vi "_DRIVER_SHARED_INI_GenerateByDriverConnectorPane.vi"() -> ()   [LabVIEW 2020]
doc: "Generate File \"_HW-Configuration_.ini\" by file [...]_driver.vi This generate the INPUT SUBSECTION using controls linked in connector pane."
uses:
  TYPEDEF/_DRIVER_SHARED_TYPEDEF_INI-Method.ctl
panel:
  in  "Path of [...]_driver.vi":path=path "C:/UG-WORK/_DRIVER_/LV2020/NI9205/NI9205_driver.vi"
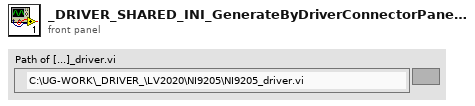
[diagram p1: front panel]
types:
  T1 = typedef "_DRIVER_SHARED_TYPEDEF_INI-Method.ctl" = enum16{"OPEN/CREATE", "READ", "WRITE", "CLOSE", "NO_OP"}
  T2 = typedef "_DRIVER_SHARED_TYPEDEF_StringControlVaviables.ctl" = cluster{"Ctrl Var Name":string, "String Ctrl Var Value":string}
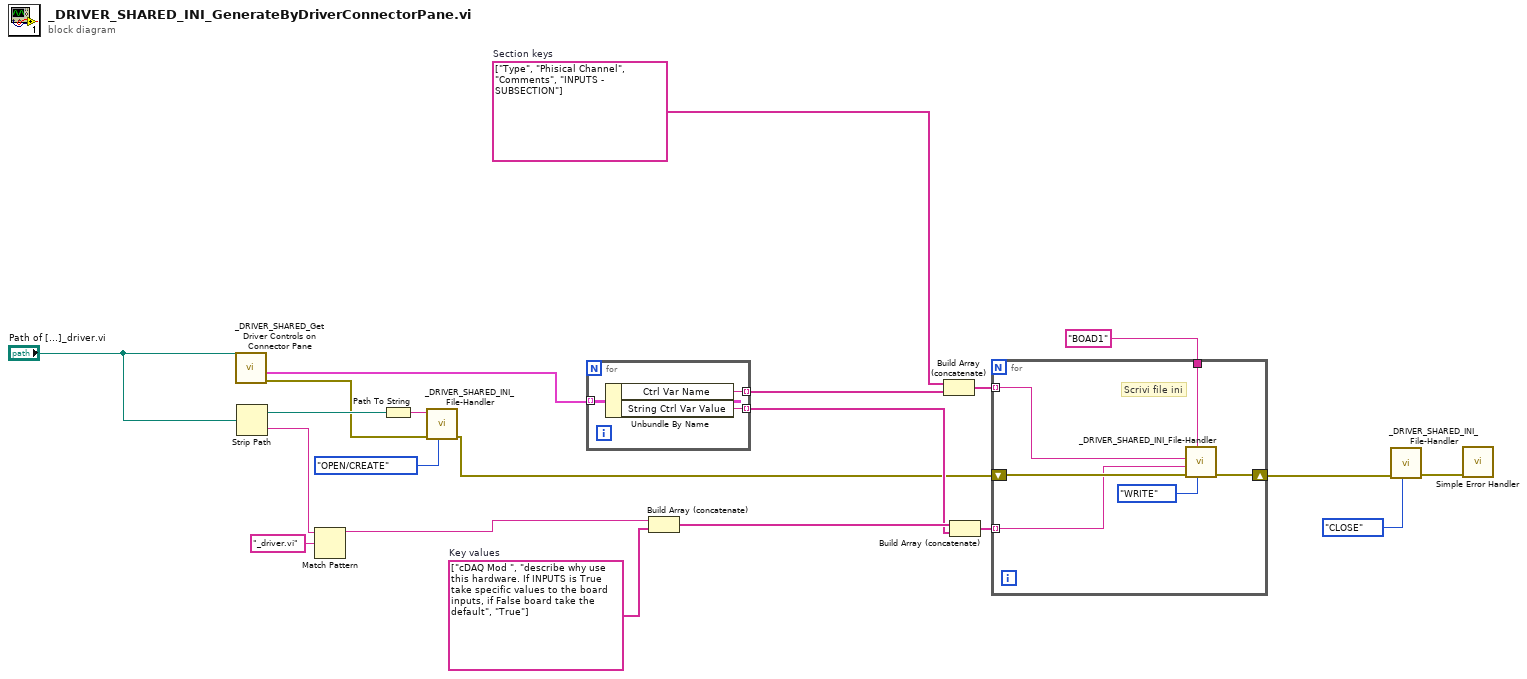
[diagram p0: block diagram]
diagram:
  w15 = string[] ["cDAQ Mod ", "describe why use this hardware. If INPUTS is True take specific values to the board inputs, if False board take the default", "True"]  # Key values
  w12 = string[] ["Type", "Phisical Channel", "Comments", "INPUTS - SUBSECTION"]  # Section keys
  n1 = call "_DRIVER_SHARED_Get Driver Controls on Connector Pane.vi"("Path of [...]_driver.vi"="Path of [...]_driver.vi") -> ("error out"=w5:errorcluster, "String Control Variables"=w4:T2[])  [unwired: 7 in, 2 out]
  n2 = Strip Path(path="Path of [...]_driver.vi") -> (stripped path=w20:path, name=w17:string)
  n3 = Match Pattern(string=w17, regular expression="_driver.vi") -> (before substring=w14:string)  [unwired: 1 in, 3 out]
  n4 = Path To String(path=w20) -> (string=w19:string)
  n5 = call "_DRIVER_SHARED_INI_File-Handler.vi"("INI-FileMethod"=_DRIVER_SHARED_TYPEDEF_INI-Method."OPEN/CREATE", "error in (no error)"=w5, "Path File"=w19) -> ("error out"=w1:errorcluster)  [unwired: 6 in, 2 out]
  n6 = for {
    tunnel: w4 -> [w24] mode=indexing
    tunnel: [w23] -> w3 mode=indexing
    tunnel: [w22] -> w2 mode=indexing
    n7 = Unbundle By Name(w24) -> ("Ctrl Var Name"=w23:string, "String Ctrl Var Value"=w22:string)
  }
  n8 = Build Array (concatenate)(w14, w15) -> (w10:string[])
  n9 = Build Array (concatenate)(w12, w3) -> (w13:string[])
  n10 = Build Array (concatenate)(w10, w2) -> (w11:string[])
  n11 = for {
    tunnel: w13 -> [w27] mode=indexing
    tunnel: w11 -> [w26] mode=indexing
    tunnel: "BOAD1" ("section IN") -> [w29]
    shift-right: [w25] -> w8
    shift-left: w1 -> [w28]
    # "Scrivi file ini"
    n12 = call "_DRIVER_SHARED_INI_File-Handler.vi"("INI-FileMethod"=_DRIVER_SHARED_TYPEDEF_INI-Method."WRITE", "section IN"=w29, "error in (no error)"=w28, "Value to write"=w26, "key IN"=w27) -> ("error out"=w25:errorcluster)  [unwired: 4 in, 2 out]
  }
  n13 = call "_DRIVER_SHARED_INI_File-Handler.vi"("INI-FileMethod"=_DRIVER_SHARED_TYPEDEF_INI-Method."CLOSE", "error in (no error)"=w8) -> ("error out"=w7:errorcluster)  [unwired: 7 in, 2 out]
  n14 = call <vilib>:"Simple Error Handler.vi"("error in (no error)"=w7) -> ()  [unwired: 4 in, 5 out]
